vi "Navigate.vi"(1 "Pathfinding Settings":T1={"Movement Settings"={"Arrival Tolerance (m)"=0.05, "Closeness Threshold (m)"=0.5, "Pit Obstacle Radius (m)"=0.5, "Pit Locations"=[]}, "Dead Zone"=0.75, "Max Moves"=2.0, "Move Segment Length (m)"=0.2, "Path Cost Weights"={"Length Weight"=1.0, "Angle Weight"=0.0, "Angle Error Weight"=75.0, "Angle Error Threshold"=1.04, "Per Move Penalty"=0.05, "Closeness Weight"=100.0, "Too Short Penalty"=100.0, "Too Short Threshold"=1.5}, "Desperation - Reduction Per Attempt (Ratio)"=0.9, "Desperation - Max Attempts"=1, "Log All Move Points"=FALSE, "Intermediate Position Grids"=[{"x1"=0.0, "x2"=1.75, "resolution"=0.5}, {"x1"=1.75, "x2"=4.5, "resolution"=0.5}]}, 2 "Move Type":T5(ring)) -> ()   [LabVIEW 2015, in "Navigation2017.lvlib"]
uses:
  Navigation2017.lvlib
  PathfindingSettings.ctl
  MovementSettings.ctl
  PathCostWeights.ctl
  IntermediatePositionGrids.ctl
  Vector.ctl
  LocalizationStatus.ctl
  PathOfMoves.ctl
  Move.ctl
  Navigation2017-util.lvlib
panel:
  out "Pathfinding Loop Count":i32=15
  in  "Reached Next Path Point Threshold Distance (m)":dbl(knob)=0.3118526382006231 scale=0.0..1.0
  in  "Robot Speed":dbl(slide)=1.0 scale=0.0..1.0
  in  "Dead Reckoning Move Distance (m)":dbl(knob)=1.4397205209376083 scale=0.5..4.0
  in  "Turning Radius (m)":dbl(knob)=1.793514692666042 scale=0.75..4.0
  # "NOTE: Log All Move Points is ignored and\nautomatically switched off."
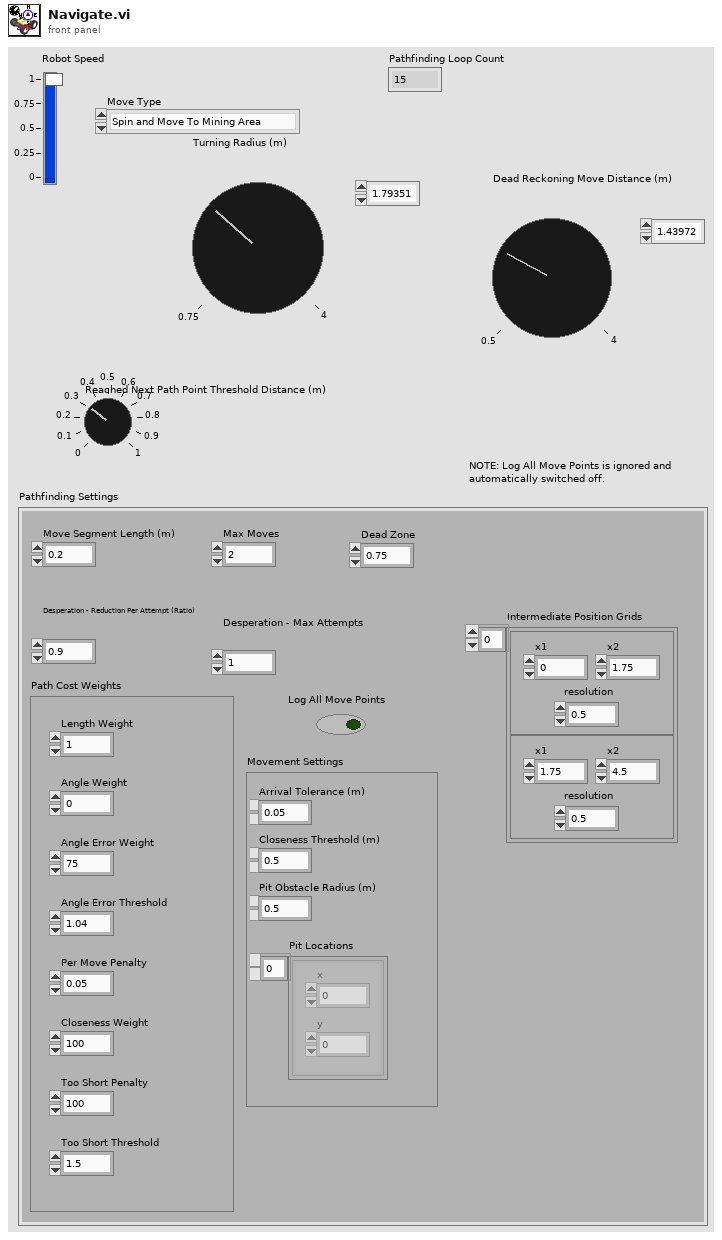
[diagram p1: front panel]
types:
  T1 = typedef "Navigation2017.lvlib/PathfindingSettings.ctl" = cluster{"Movement Settings":T2, "Dead Zone":dbl, "Max Moves":dbl, "Move Segment Length (m)":dbl, "Path Cost Weights":T3, "Desperation - Reduction Per Attempt (Ratio)":dbl, "Desperation - Max Attempts":i16, "Log All Move Points":bool, "Intermediate Position Grids":T4}
  T2 = typedef "Navigation2017.lvlib/MovementSettings.ctl" = cluster{"Arrival Tolerance (m)":dbl, "Closeness Threshold (m)":dbl, "Pit Obstacle Radius (m)":dbl, "Pit Locations":cluster{"x":dbl, "y":dbl}[]}
  T3 = typedef "Navigation2017.lvlib/PathCostWeights.ctl" = cluster{"Length Weight":dbl, "Angle Weight":dbl, "Angle Error Weight":dbl, "Angle Error Threshold":dbl, "Per Move Penalty":dbl, "Closeness Weight":dbl, "Too Short Penalty":dbl, "Too Short Threshold":dbl}
  T4 = typedef "Navigation2017.lvlib/IntermediatePositionGrids.ctl" = cluster{"x1":dbl, "x2":dbl, "resolution":dbl}[]
  T5 = enum16{"Spin and Move To Mining Area", "Move To Collector Trough", "Move To Mining Area"}
  T6 = typedef "Navigation2017.lvlib/Vector.ctl" = cluster{"x":dbl, "y":dbl, "angle":dbl}
  T7 = typedef "LocalizationStatus.ctl" = cluster{"x":dbl, "y":dbl, "angle":dbl, "valid":bool, "lastUpdatedTime":dbl}
  T8 = typedef "Navigation2017.lvlib/PathOfMoves.ctl" = cluster{"Dest Angle Error":dbl, "Dest Angle Considered":bool, "Moves":T9[]}
  T9 = typedef "Navigation2017.lvlib/Move.ctl" = cluster{"Did Reach Dest":bool, "Did Collide":bool, "Sum of Angle Changes (rad)":dbl, "Move Length (m)":dbl, "Closeness Sum":dbl, "Positions Along Move":T6[], "Moved Fwd":bool}
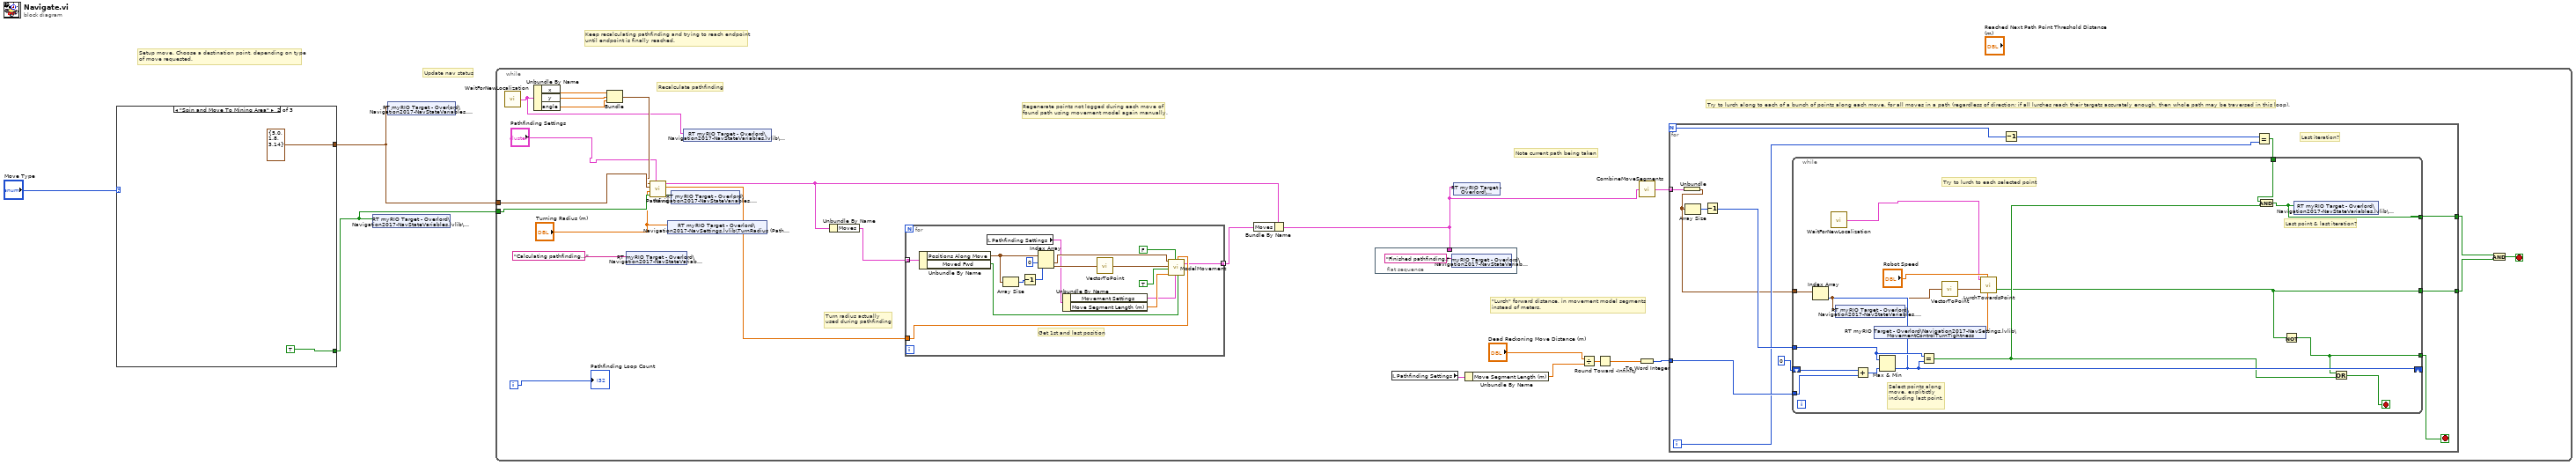
[diagram p0: block diagram]
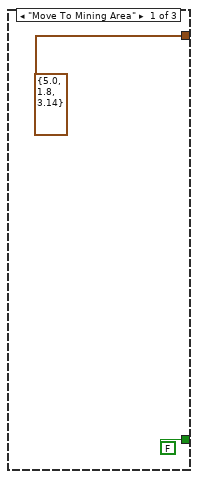
[diagram p2: hidden frame]
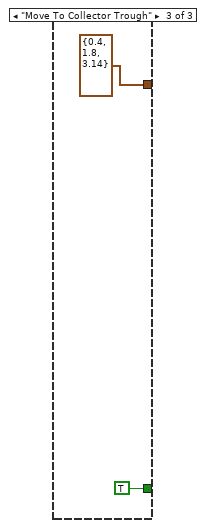
[diagram p3: hidden frame]
diagram:
  # "Keep recalculating pathfinding and trying to reach endpoint\nuntil endpoint is finally reached."
  # "Update nav status"
  # "Setup move. Choose a destination point, depending on type\nof move requested."
  n1 = case shown="\"Spin and Move To Mining Area\"" "Move Type" {
    tunnel: [T6 {"x"=5.0, "y"=1.8, "angle"=3.14} ("Vector") T6 {"x"=5.0, "y"=1.8, "angle"=3.14} ("Vector") T6 {"x"=0.4, "y"=1.8, "angle"=3.14} ("Vector")] -> w2
    tunnel: [FALSE TRUE TRUE] -> w1
    frame "Move To Mining Area" {
    }
    frame "Spin and Move To Mining Area" {
    }
    frame "Move To Collector Trough" {
    }
  }
  n2 = shared-variable "RT myRIO Target - Overlord\\Navigation2017-NavStateVariables.lvlib\\SpecifyingEndAngle"(w1) -> ()  [unwired: 1 in, 1 out]
  n3 = shared-variable "RT myRIO Target - Overlord\\Navigation2017-NavStateVariables.lvlib\\DestinationPoint"(w2) -> ()  [unwired: 1 in, 1 out]
  n4 = while {
    tunnel: w2 -> [w35]
    tunnel: w1 -> [w34]
    i -> [w36]
    stop <- w23 stop-if-true
    # "Try to lurch along to each of a bunch of points along each move, for all moves in a path (regardless of direction; if all lurches reach their targets accurately enough, then whole path may be traversed in this loop)."
    # "Turn radius actually\nused during pathfinding"
    # "Regenerate points not logged during each move of\nfound path using movement model again manually."
    # "\"Lurch\" forward distance, in movement model segments\ninstead of meters."
    # "Note current path being taken"
    # "Recalculate pathfinding"
    n5 = call "WaitForNewLocalization.vi"() -> ("Localization Status"=w17:T7)
    n6 = Unbundle By Name(w17) -> ("x"=w20:dbl, "y"=w19:dbl, "angle"=w18:dbl)
    n7 = Bundle("x"=w20, "y"=w19, "angle"=w18) -> (w21:cluster{"x":dbl, "y":dbl, "angle":dbl})  [unwired: 1 in]
    n8 = shared-variable "RT myRIO Target - Overlord\\Navigation2017-NavStateVariables.lvlib\\CurrNavStage"("Calculating pathfinding..." ("CurrNavStage")) -> ()  [unwired: 1 in, 1 out]
    n9 = call "Pathfind.vi"("Pathfinding Settings"="Pathfinding Settings", "Specified End Angle"=w34, "Turn Radius (m)"="Turning Radius (m)", "Destination"=w35, "Start Vector"=w21) -> ("Desperation Used"=w33:bool, "Used Turn Radius (m)"=w16:dbl, "Best Path"=w12:T8)  [unwired: 2 out]
    n10 = shared-variable "RT myRIO Target - Overlord\\Navigation2017-NavSettings.lvlib\\TurnRadius (Path Modeling)"("Turning Radius (m)") -> ()  [unwired: 1 in, 1 out]
    n11 = shared-variable "RT myRIO Target - Overlord\\Navigation2017-NavStateVariables.lvlib\\UsedDesperation"(w33) -> ()  [unwired: 1 in, 1 out]
    n12 = shared-variable "RT myRIO Target - Overlord\\Navigation2017-NavStateVariables.lvlib\\PathfindingStartPosition"(w17) -> ()  [unwired: 1 in, 1 out]
    n13 = Unbundle By Name(w12) -> ("Moves"=w15:T9[])
    n14 = for {
      tunnel: w16 -> [w53]
      tunnel: w15 -> [w52] mode=indexing
      tunnel: [w42] -> w14 mode=indexing
      # "Get 1st and last position"
      n15 = Unbundle By Name(w52) -> ("Positions Along Move"=w40:T6[], "Moved Fwd"=w51:bool)
      n16 = local read "Pathfinding Settings"() -> (w45:T1)
      n17 = Array Size(array=w40) -> (size(s)=w39:i32)
      n18 = Decrement(x=w39) -> (x-1=w38:i32)
      n19 = Index Array(array=w40, index #1=0 ("index"), index #2=w38) -> (element #1=w49:T6, element #2=w47:T6)
      n20 = Unbundle By Name(w45) -> ("Movement Settings"=w43:T2, "Move Segment Length (m)"=w44:dbl)
      n21 = call "VectorToPoint.vi"("Vector"=w47) -> ("Point"=w48:cluster{"x":dbl, "y":dbl})
      n22 = call "ModelMovement.vi"("Start Vector"=w49, "Destination"=w48, "Log All Points"=TRUE, "Segment Length (m)"=w44, "Do Force Direction"=FALSE, "Movement Settings"=w43, "Turn Radius (m)"=w53, "Force Direction Forward (If Forcing)"=w51) -> ("Move"=w42:T9)  [unwired: 10 in, 1 out]
    }
    n23 = Bundle By Name(cluster=w12, "Moves"=w14) -> (w11:T8)
    n24 = flat-sequence {
      tunnel: w11 -> [_]
      frame #0 {
        n25 = shared-variable "RT myRIO Target - Overlord\\Navigation2017-NavStateVariables.lvlib\\CurrNavStage"("Finished pathfinding." ("CurrNavStage")) -> ()  [unwired: 1 in, 1 out]
      }
    }
    n26 = local read "Pathfinding Settings"() -> (w28:T1)
    n27 = shared-variable "RT myRIO Target - Overlord\\Navigation2017-NavStateVariables.lvlib\\CurrPath"(w11) -> ()  [unwired: 1 in, 1 out]
    n28 = Unbundle By Name(w28) -> ("Move Segment Length (m)"=w29:dbl)
    n29 = Divide(x="Dead Reckoning Move Distance (m)", y=w29) -> (x/y=w31:dbl)
    n30 = Round Toward -Infinity(1:w31) -> (0:w26:dbl)
    n31 = call "CombineMoveSegments.vi"("Path"=w11) -> ("Combined Moves & Positions"=w22:cluster{T6[]}[])
    n32 = To Word Integer(number=w26) -> (16bit integer=w27:i16)
    n33 = for {
      N -> [w61]
      tunnel: w27 -> [w66]
      tunnel: [w57] -> w25
      tunnel: [w56] -> w24
      tunnel: w22 -> [w55] mode=indexing
      i -> [w59]
      stop <- w62 stop-if-true
      # "Last iteration?"
      n34 = Unbundle(w55) -> (w54:T6[])
      n35 = Array Size(array=w54) -> (size(s)=w64:i32)
      n36 = Decrement(x=w64) -> (x-1=w63:i32)
      n37 = Decrement(x=w61) -> (x-1=w60:i32)
      n38 = Equal?(x=w60, y=w59) -> (x = y?=w58:bool)
      n39 = while {
        shift-right: [w78] -> _
        shift-left: i16 0 -> [w82]
        tunnel: w66 -> [w83]
        tunnel: w63 -> [w80]
        tunnel: w54 -> [w77]
        tunnel: [w74] -> w62
        tunnel: w58 -> [w72]
        tunnel: [w71] -> w57
        tunnel: [w67] -> w56
        stop <- w75 stop-if-true
        # "Select points along\nmove, explitictly including last point."
        # "Last point & last iteration?"
        # "Try to lurch to each selected point"
        n40 = call "WaitForNewLocalization.vi"() -> ("Localization Status"=w68:T7)
        n41 = Add(x=w82, y=w83) -> (x+y=w81:i32)
        n42 = shared-variable "RT myRIO Target - Overlord\\Navigation2017-NavSettings.lvlib\\MovementControlTurnTightness"() -> (w69:dbl)  [unwired: 1 in, 1 out]
        n43 = Max & Min(x=w80, y=w81) -> (min(x,y)=w78:i32)  [unwired: 1 out]
        n44 = Index Array(array=w77, index=w78) -> (element=w70:T6)
        n45 = shared-variable "RT myRIO Target - Overlord\\Navigation2017-NavStateVariables.lvlib\\NextPointOnPath"(w70) -> ()  [unwired: 1 in, 1 out]
        n46 = Equal?(x=w80, y=w78) -> (x = y?=w73:bool)
        n47 = call "VectorToPoint.vi"("Vector"=w70) -> ("Point"=w79:cluster{"x":dbl, "y":dbl})
        n48 = call "LurchTowardsPoint.vi"("Turning Radius (m) \n(Goes into Dillons' Movement Control)"=w69, "Robot Speed"="Robot Speed", "Dest. Point"=w79, "Curr Localization Status"=w68) -> ("Within Tolerance of Dest (DEPRECATED AND BROKEN)"=w67:bool)  [unwired: 2 in, 1 out]
        n49 = And(x=w72, y=w73) -> (x .and. y?=w71:bool)
        n50 = Not(x=w67) -> (.not. x?=w74:bool)
        n51 = shared-variable "RT myRIO Target - Overlord\\Navigation2017-NavStateVariables.lvlib\\NextPointIsDestination"(w71) -> ()  [unwired: 1 in, 1 out]
        n52 = Or(x=w74, y=w73) -> (x .or. y?=w75:bool)
      }
    }
    n53 = And(x=w25, y=w24) -> (x .and. y?=w23:bool)
    "Pathfinding Loop Count" <- w36
  }
